vi "InitCfg.vi"(8 "error in (no error)":errorcluster, 9 "Cfg File path":path=path "C:/Users/Public/Documents/OU PAARD/mmWave_RF_Scanner/SupportFiles/mmWaveVXMConfig.ini") -> (0 "error out":errorcluster, 1 "Serial Port":cluster{"Addr":string, "Enable":bool}={"Addr"="COM3", "Enable"=FALSE}, 3 "VXMCfg out":refnum<class "VXMCfg.lvclass">)   [LabVIEW 2018, in "VXMCfg.lvclass"]
uses:
  VXMCfg.lvclass
  VXMCfg.ctl
  sub-syst.n.ctl
  VXMCfg.lvclass/VXMCfg.ctl
panel:
  in  "VXM Properties":T1={"sub-syst1"={"Addr"="COM3", "Enable"=FALSE, "X scale eng./step"=0.0125, "Y scale eng./step"=0.00635, "Z scale eng./step"=0.00635, "T scale eng./step"=1.0, "X units"="deg", "Y units"="mm", "Z units"="mm", "T units"="", "X Jog"=1.0, "Y Jog"=1.0, "Z Jog"=1.0, "T Jog"=1.0, "X-1 Name"="RT1", "Y-2 Name"="BS2", "Z-3 Name"="BS1", "T-4 Name"="", "VXM (1-4)"=3}, "sub-syst2"={"Addr"="COM4", "Enable"=FALSE, "X scale eng./step"=0.00635, "Y scale eng./step"=0.00635, "Z scale eng./step"=0.0125, "T scale eng./step"=0.0125, "X units"="mm", "Y units"="mm", "Z units"="deg", "T units"="deg", "X Jog"=1.0, "Y Jog"=1.0, "Z Jog"=1.0, "T Jog"=1.0, "X-1 Name"="RT2", "Y-2 Name"="BS3", "Z-3 Name"="BS4", "T-4 Name"="RT3", "VXM (1-4)"=4}, "sub-syst3"={"Addr"="COM5", "Enable"=FALSE, "X scale eng./step"=0.00635, "Y scale eng./step"=0.0125, "Z scale eng./step"=1.0, "T scale eng./step"=1.0, "X units"="mm", "Y units"="deg", "Z units"="", "T units"="", "X Jog"=1.0, "Y Jog"=1.0, "Z Jog"=1.0, "T Jog"=1.0, "X-1 Name"="BS5", "Y-2 Name"="RT4", "Z-3 Name"="", "T-4 Name"="", "VXM (1-4)"=2}}
  # ".00025 in/step\ncalculates to \n.00635 mm/step"
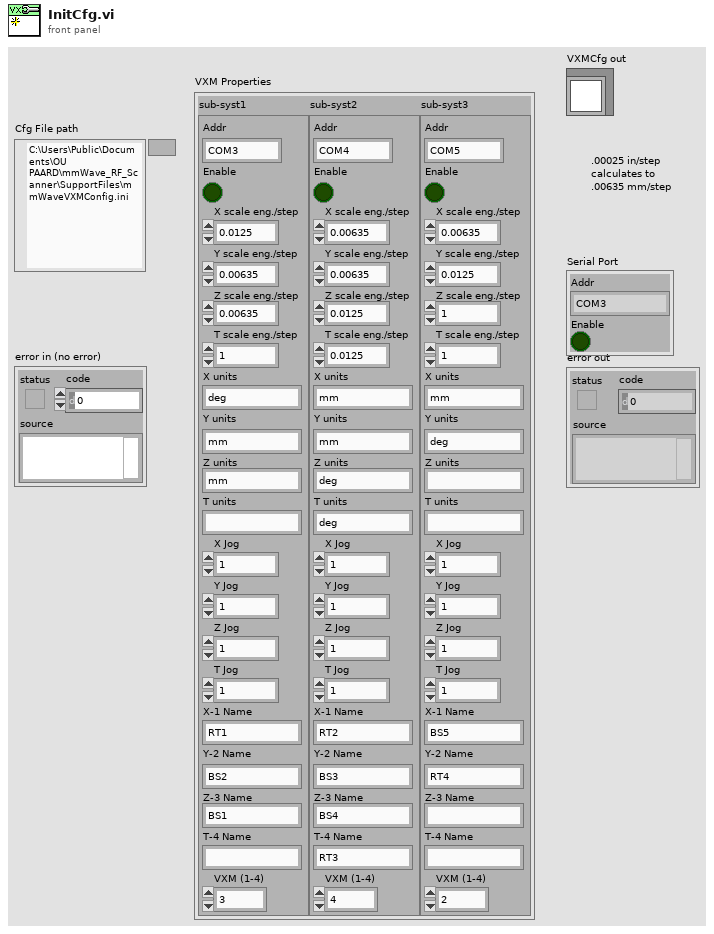
[diagram p1: front panel]
types:
  T1 = typedef "VXMCfg.ctl" = cluster{"sub-syst1":T2, "sub-syst2":T2, "sub-syst3":T2}
  T2 = typedef "sub-syst.n.ctl" = cluster{"Addr":string, "Enable":bool, "X scale eng./step":dbl, "Y scale eng./step":dbl, "Z scale eng./step":dbl, "T scale eng./step":dbl, "X units":string, "Y units":string, "Z units":string, "T units":string, "X Jog":dbl, "Y Jog":dbl, "Z Jog":dbl, "T Jog":dbl, "X-1 Name":string, "Y-2 Name":string, "Z-3 Name":string, "T-4 Name":string, "VXM (1-4)":i32}
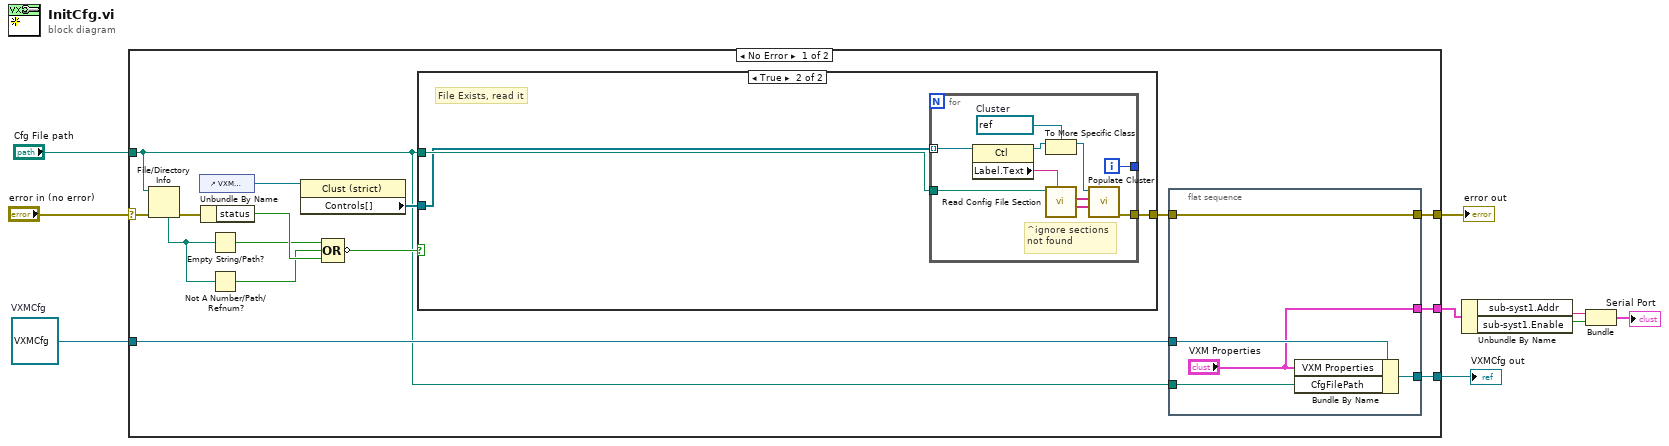
[diagram p0: block diagram]
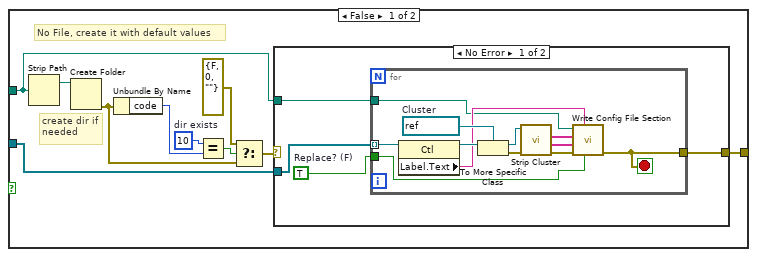
[diagram p2: hidden frame]
diagram:
  w7 = refnum<class "VXMCfg.lvclass"> refnum  # VXMCfg
  n1 = case shown="No Error" "error in (no error)" {
    selector: "error in (no error)" -> [w14 w71]
    tunnel: [w13 w71] -> w6
    tunnel: [w15 w70] -> w5
    tunnel: w7 -> [w16 w70]
    tunnel: "Cfg File path" -> [w12 _]
    tunnel: [w10 _] -> w4
    frame No Error {
      n2 = File/Directory Info(path=w12, error in=w14) -> (error out=w20:errorcluster, resolved path=w17:path)  [unwired: 5 out]
      n3 = control-ref of="VXM Properties"() -> (w11:refnum<vi>)
      n4 = Unbundle By Name(w20) -> ("status"=w21:bool)
      n5 = Empty String/Path?(string/path=w17) -> (empty?=w18:bool)
      n6 = Not A Number/Path/Refnum?(number/path/refnum=w17) -> (NaN/Path/Refnum?=w19:bool)
      n7 = property class="Clust (strict)"(reference=w11) -> ("Controls[]"=w22:refnum<vi>[])  [unwired: 1 in, 2 out]
      n8 = Compound Arithmetic op=OR(w18, w19, w21) -> (invert w23:bool)
      n9 = case shown="True" w23 {
        tunnel: w12 -> [w37 w59]
        tunnel: w22 -> [w39 w58]
        tunnel: [w38 w57] -> w24
        frame False {
          w32 = 10  # dir exists
          # "create dir if\nneeded"
          # "No File, create it with default values"
          n10 = Strip Path(path=w37) -> (stripped path=w34:path)  [unwired: 1 out]
          n11 = Create Folder(path (use dialog)=w34) -> (error out=w33:errorcluster)  [unwired: 2 in, 2 out]
          n12 = Unbundle By Name(w33) -> ("code"=w36:i32)
          n13 = Equal?(x=w32, y=w36) -> (x = y?=w35:bool)
          n14 = Select(t=errorcluster {"status"=FALSE, "code"=0, "source"=""}, s=w35, f=w33) -> (s? t:f=w30:errorcluster)
          n15 = case shown="No Error" w30 {
            selector: w30 -> [_ w56]
            tunnel: w39 -> [w43 _]
            tunnel: [w41 w56] -> w38
            tunnel: w37 -> [w40 _]
            frame No Error {
              w42 = TRUE  # Replace? (F)
              n16 = for {
                tunnel: w43 -> [w48] mode=indexing
                tunnel: [w49] -> w41
                tunnel: w42 -> [w45]
                tunnel: w40 -> [w44]
                stop <- w49 stop-if-true
                w55 = refnum<vi> refnum  # Cluster
                n17 = property class="Ctl"(reference=w48) -> (reference out=w47:refnum<vi>, "Label.Text"=w46:string)  [unwired: 1 in, 1 out]
                n18 = To More Specific Class(target class=w55, reference=w47) -> (specific class reference=w54:refnum<vi>, error out=w51:errorcluster)  [unwired: 1 in]
                n19 = call "Strip Cluster.vi"("error in (no error)"=w51, "Cluster Refnum"=w54) -> ("error out"=w50:errorcluster, "Values"=w52:string[], "Keys"=w53:string[])  [unwired: 6 in, 1 out]
                n20 = call "Write Config File Section.vi"("Replace? (F)"=w45, "Section"=w46, "error in"=w50, "Values"=w52, "Keys"=w53, "INI path"=w44) -> ("error out"=w49:errorcluster)  [unwired: 5 in]
              }
            }
            frame Error {
            }
          }
        }
        frame True {
          # "File Exists, read it"
          n21 = for {
            tunnel: w58 -> [w69] mode=indexing
            tunnel: w59 -> [w67]
            tunnel: [w64] -> w57
            tunnel: [w60] -> _
            i -> [w60]
            w63 = refnum<vi> refnum  # Cluster
            # "^ignore sections\nnot found"
            n22 = property class="Ctl"(reference=w69) -> (reference out=w62:refnum<vi>, "Label.Text"=w68:string)  [unwired: 1 in, 1 out]
            n23 = To More Specific Class(target class=w63, reference=w62) -> (specific class reference=w61:refnum<vi>)  [unwired: 1 in, 1 out]
            n24 = call "Read Config File Section.vi"("Section"=w68, "appended path"=w67) -> ("Values"=w65:string[], "Keys"=w66:string[])  [unwired: 7 in, 1 out]
            n25 = call "Populate Cluster.vi"("Values"=w65, "Keys"=w66, "Clust Refnum"=w61) -> ("error out"=w64:errorcluster)  [unwired: 7 in, 1 out]
          }
        }
      }
      n26 = flat-sequence {
        tunnel: w12 -> [w29]
        tunnel: w16 -> [w28]
        tunnel: [w27] -> w15
        tunnel: [w26] -> w13
        tunnel: w24 -> [w26]
        tunnel: ["VXM Properties"] -> w10
        frame #0 {
          n27 = Bundle By Name(cluster=w28, "VXM Properties"="VXM Properties", "CfgFilePath"=w29) -> (w27:refnum<class "VXMCfg.lvclass">)
        }
      }
    }
    frame Error {
    }
  }
  "error out" <- w6
  "VXMCfg out" <- w5
  n28 = Unbundle By Name(w4) -> ("sub-syst1.Addr"=w2:string, "sub-syst1.Enable"=w3:bool)
  n29 = Bundle("Addr"=w2, "Enable"=w3) -> (→"Serial Port":cluster{"Addr":string, "Enable":bool})  [unwired: 1 in]
